vi "% span to Arduino Signal v1.vi"(2 "% span":dbl=100.0 format="%.2f") -> (0 "Output":dbl=100.0 format="%.2f")   [LabVIEW 2012]
panel:
  in  "Minimum Output":dbl format="%.2f"
  in  "Maximum Output":dbl=100.0 format="%.2f"
  # "% span to Output"
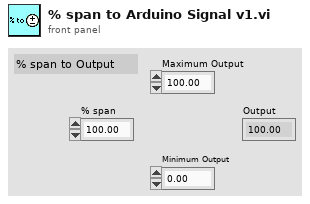
[diagram p1: front panel]
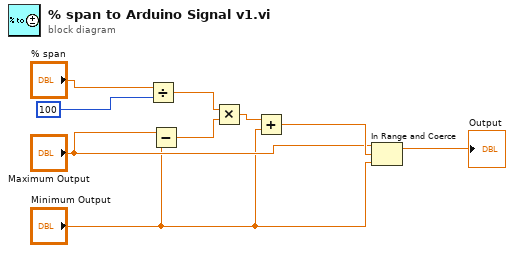
[diagram p0: block diagram]
diagram:
  n1 = Divide(x="% span", y=100) -> (x/y=w7:dbl)
  n2 = Subtract(x="Maximum Output", y="Minimum Output") -> (x-y=w6:dbl)
  n3 = Multiply(x=w7, y=w6) -> (x*y=w5:dbl)
  n4 = Add(x=w5, y="Minimum Output") -> (x+y=w4:dbl)
  n5 = In Range and Coerce(upper limit="Maximum Output", x=w4, lower limit="Minimum Output") -> (coerced(x)=→"Output":dbl)  [unwired: 1 out]
